vi "Calculate Padding Buffer Size.vi"(10 "LP  F":dbl=0.001 format="%#_6p", 11 "Array size":i32) -> (1 "Last element":i32, 2 "First element":i32, 3 "Buffer size":i32)   [LabVIEW 2016]
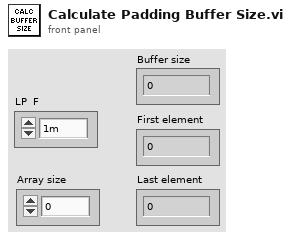
[diagram p1: front panel]
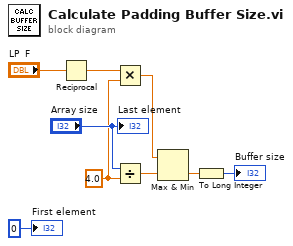
[diagram p0: block diagram]
diagram:
  w5 = 4.0 ("y")
  n1 = Reciprocal(x="LP  F") -> (1/x=w7:dbl)
  n2 = Multiply(x=w7, y=w5) -> (x*y=w8:dbl)
  n3 = Divide(x="Array size", y=w5) -> (x/y=w4:dbl)
  n4 = Max & Min(x=w8, y=w4) -> (min(x,y)=w3:dbl)  [unwired: 1 out]
  n5 = To Long Integer(number=w3) -> (32bit integer=→"Buffer size":i32)
  "Last element" <- "Array size"
  "First element" <- 0 ("First element")
